vi "Ctrls - Set Display State of all FP Controls.vi"(0 "VI Path":path, 3 "Display State":T1) -> ()   [LabVIEW 2011]
uses:
  Control - Display State.ctl
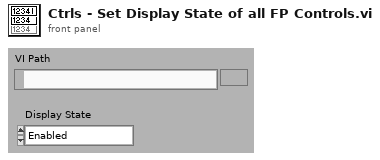
[diagram p1: front panel]
types:
  T1 = typedef "Control - Display State.ctl" = enum16{"Enabled", "Disabled", "Disabled and Grayed"}
  T2 = enum32{"existing file", "new file", "new or existing file", "existing dir", "new dir", "new or existing dir", "existing file (use LLBs)", "new file (use LLBs)", "new or existing file (use LLBs)", "new or existing file or directory (use LLBs)"}
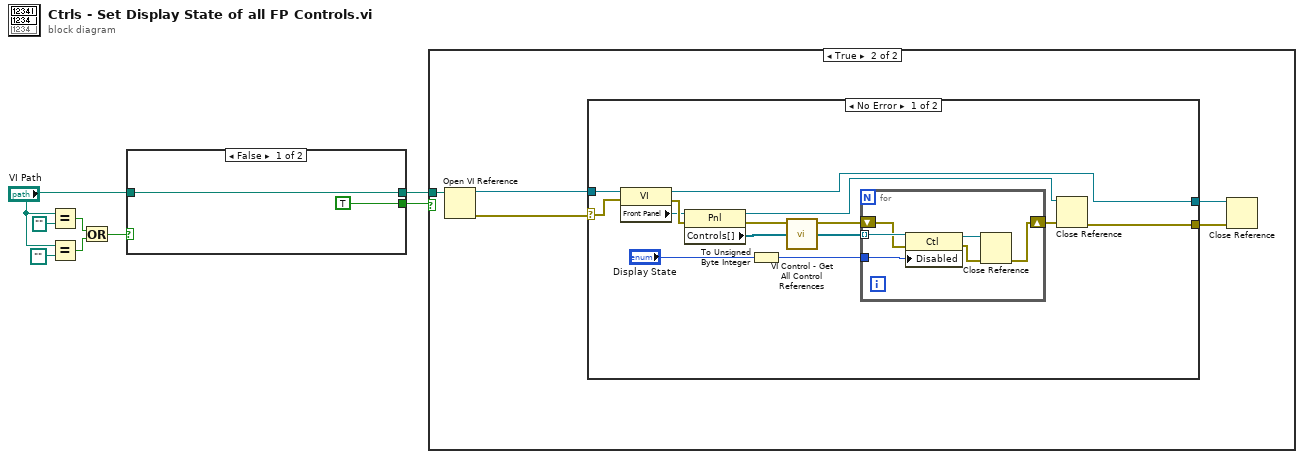
[diagram p0: block diagram]
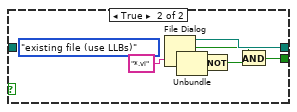
[diagram p4: hidden frame]
diagram:
  n1 = Equal?(x="VI Path", y=path "") -> (x = y?=w6:bool)
  n2 = Equal?(x="VI Path", y=path "") -> (x = y?=w5:bool)
  n3 = Or(x=w6, y=w5) -> (x .or. y?=w4:bool)
  n4 = case shown="False" w4 {
    tunnel: "VI Path" -> [w10 _]
    tunnel: [w10 w16] -> w2
    tunnel: [TRUE w12] -> w1
    frame False {
    }
    frame True {
      (unwired) T2."existing file (use LLBs)" ("select mode (2)")
      n5 = File Dialog(6:"*.vi" ("pattern")) -> (0:w11:errorcluster, 1:w15:bool, 2:w13:bool, 3:w16:path)  [unwired: 6 in]
      n6 = Unbundle(w11) -> ()  [unwired: 3 out]
      n7 = Not(x=w15) -> (.not. x?=w14:bool)
      n8 = And(x=w13, y=w14) -> (x .and. y?=w12:bool)
    }
  }
  n9 = case shown="True" w1 {
    tunnel: w2 -> [_ w19]
    frame False {
    }
    frame True {
      n10 = Open VI Reference(vi path=w19) -> (vi reference=w20:refnum<vi>, error out=w18:errorcluster)  [unwired: 5 in]
      n11 = case shown="No Error" w18 {
        selector: w18 -> [w23 w42]
        tunnel: [w31 w42] -> w22
        tunnel: [w30 w43] -> w21
        tunnel: w20 -> [w28 w43]
        frame No Error {
          n12 = property class="VI"(reference=w28, error in=w23) -> (reference out=w30:refnum<vi>, error out=w35:errorcluster, "Front Panel"=w29:refnum<vi>)
          n13 = property class="Pnl"(reference=w29, error in=w35) -> (reference out=w32:refnum<vi>, error out=w34:errorcluster, "Controls[]"=w27:refnum<vi>[])
          n14 = To Unsigned Byte Integer(number="Display State") -> (unsigned 8bit integer=w24:u8)
          n15 = call "VI Control - Get All Control References.vi"("Control References - Top Level"=w27) -> ("Control References - Complete"=w26:refnum<vi>[])  [unwired: 12 in, 2 out]
          n16 = for {
            tunnel: w26 -> [w41] mode=indexing
            shift-right: [w37] -> w33
            shift-left: w34 -> [w40]
            tunnel: w24 -> [w36]
            n17 = property class="Ctl"(reference=w41, error in=w40, "Disabled"=w36) -> (reference out=w38:refnum<vi>, error out=w39:errorcluster)
            n18 = Close Reference(reference=w38, error in (no error)=w39) -> (error out=w37:errorcluster)
          }
          n19 = Close Reference(reference=w32, error in (no error)=w33) -> (error out=w31:errorcluster)
        }
        frame Error {
          # "Error opening reference to vi"
        }
      }
      n20 = Close Reference(reference=w21, error in (no error)=w22) -> ()  [unwired: 1 out]
    }
  }
